vi "Solution.vi"() -> ()   [LabVIEW 2020]
uses:
  <vilib>/Utility/file.llb/Read Delimited Spreadsheet (I64).vi
panel:
  out "result":i32
  in  "data?":bool
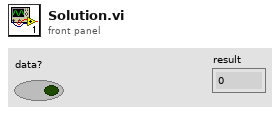
[diagram p1: front panel]
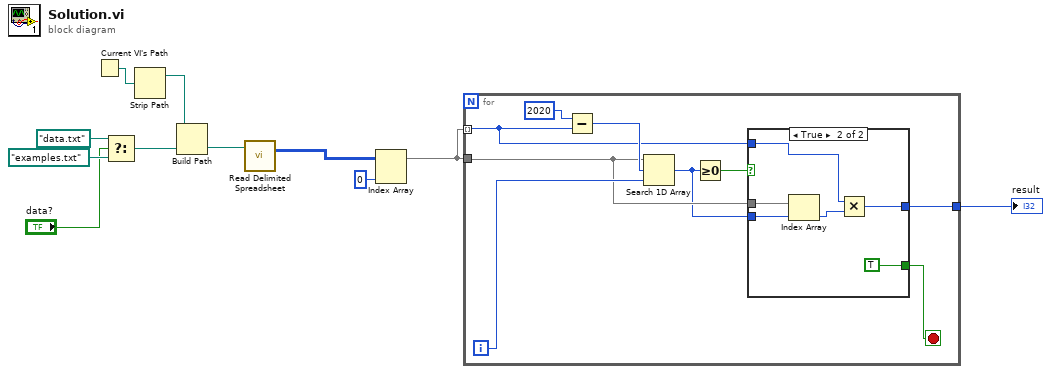
[diagram p0: block diagram]
diagram:
  n1 = Current VI's Path() -> (path=w6:path)
  n2 = Select(t=path "data.txt", s="data?", f=path "examples.txt") -> (s? t:f=w8:path)
  n3 = Strip Path(path=w6) -> (stripped path=w5:path)  [unwired: 1 out]
  n4 = Build Path(base path=w5, name or relative path=w8) -> (appended path=w4:path)
  n5 = call-poly <vilib>:"Read Delimited Spreadsheet.vi"("file path (dialog if empty)"=w4) -> ("all rows"=w3:i64[][])  [unwired: 9 in, 5 out]
  n6 = Index Array(array=w3, index (col)=0 ("disabled index (col)")) -> (element=w2:i64[])  [unwired: 1 in]
  n7 = for {
    tunnel: w2 -> [w16]
    tunnel: w2 -> [w14] mode=indexing
    tunnel: [w13] -> w7
    i -> [w20]
    stop <- w12 stop-if-true
    n8 = Subtract(x=2020, y=w14) -> (x-y=w18:i64)
    n9 = Search 1D Array(1D array=w16, element=w18, start index (0)=w20) -> (index of element=w15:i32)
    n10 = Greater Or Equal To 0?(x=w15) -> (x >= 0?=w17:bool)
    n11 = case shown="True" w17 {
      tunnel: w16 -> [_ w27]
      tunnel: w15 -> [w21 w26]
      tunnel: w14 -> [_ w24]
      tunnel: [w21 w23] -> w13
      tunnel: [_ TRUE] -> w12
      frame False {
      }
      frame True {
        n12 = Index Array(array=w27, index=w26) -> (element=w25:i64)
        n13 = Multiply(x=w24, y=w25) -> (x*y=w23:i64)
      }
    }
  }
  "result" <- w7
